vi "MeasurementStatus.vi"(8 "error in (no error)":errorcluster, 10 "Current Measurement Idx":i32, 11 "Measurement Sequence":dbl[](array[numeric])) -> (0 "error out":errorcluster, 2 "Sequence Progress":cluster{i32[], "Y":dbl[]}[](array[cluster]))   [LabVIEW 2014]
panel:
  # "LICENSED MATERIALS – PROPERTY OF IBM\nCopyright IBM Corp. 2016,\nALL RIGHTS RESERVED"
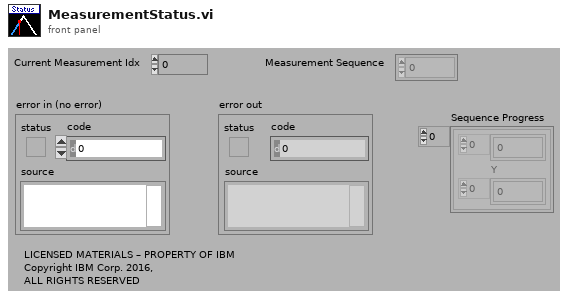
[diagram p1: front panel]
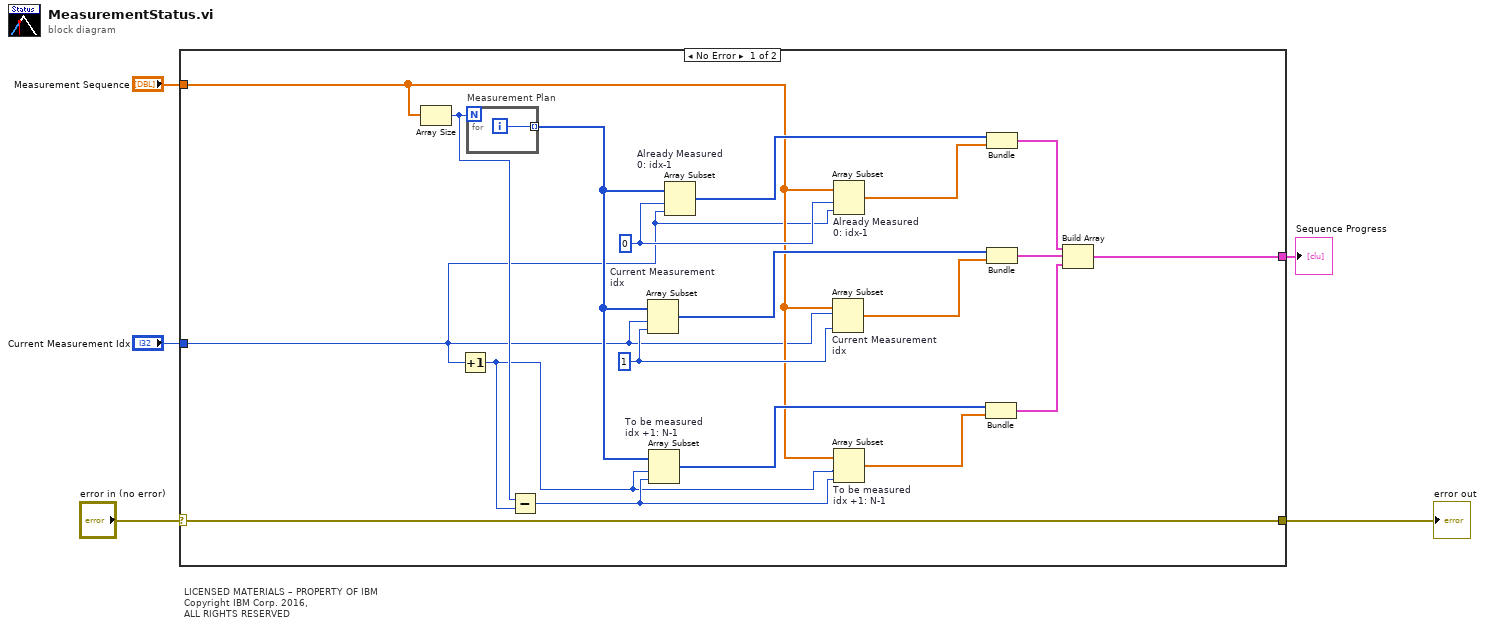
[diagram p0: block diagram]
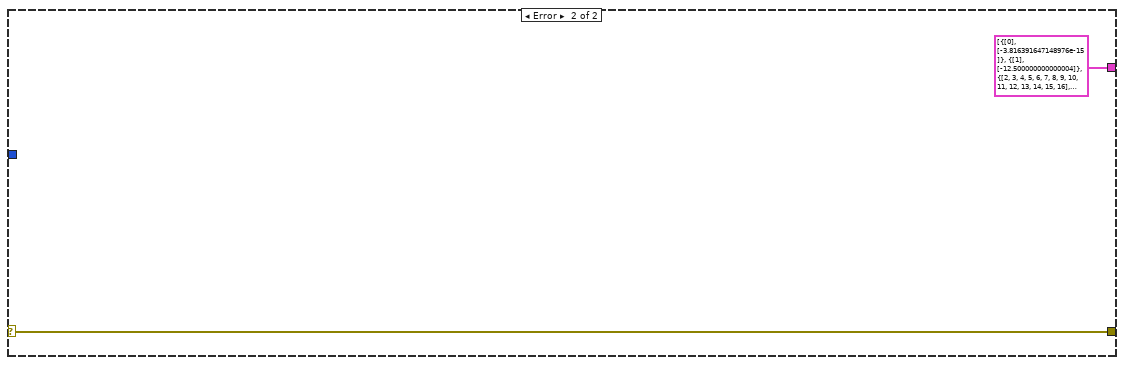
[diagram p2: hidden frame]
diagram:
  # "LICENSED MATERIALS – PROPERTY OF IBM\nCopyright IBM Corp. 2016,\nALL RIGHTS RESERVED"
  n1 = case shown="No Error" "error in (no error)" {
    selector: "error in (no error)" -> [w9 w27]
    tunnel: [w9 w27] -> w4
    tunnel: [w8 cluster{i32[], "Y":dbl[]}[] [{[0], "Y"=[-3.816391647148976e-15]}, {[1], "Y"=[-12.500000000000004]}, {[2, 3, 4, 5, 6, 7, 8, 9, 10, 11, 12, 13, 14, 15, 16], "Y"=[-25.000000000000004, -37.50000000000001, -49.99999999999999, -37.49999999999999, -24.999999999999993, -12.499999999999993, 0.0, 12.5, 25.0, 37.5, 50.0, 37.5, 24.999999999999996, 12.499999999999996, -3.816391647148976e-15]}] ("Sequence Progress 2")] -> w3
    tunnel: "Measurement Sequence" -> [w7 _]
    tunnel: "Current Measurement Idx" -> [w6 _]
    frame No Error {
      w23 = 0 ("index")
      w22 = 1 ("length")
      n2 = Array Size(array=w7) -> (size(s)=w24:i32)
      n3 = Increment(x=w6) -> (x+1=w20:i32)
      n4 = for "Measurement Plan" {
        N: w24 -> [_]
        tunnel: [w25] -> w19 mode=indexing
        i -> [w25]
      }
      n5 = Subtract(x=w24, y=w20) -> (x-y=w21:i32)
      n6 = Array Subset "Current Measurement\nidx"(array=w19, index=w6, length=w22) -> (w16:i32[])
      n7 = Array Subset "To be measured\nidx +1: N-1"(array=w19, index=w20, length=w21) -> (w14:i32[])
      n8 = Array Subset "Already Measured\n0: idx-1"(array=w19, index=w23, length=w6) -> (w18:i32[])
      n9 = Array Subset "Current Measurement\nidx"(array=w7, index=w6, length=w22) -> (w15:dbl[])
      n10 = Array Subset "Already Measured\n0: idx-1"(array=w7, index=w23, length=w6) -> (w17:dbl[])
      n11 = Array Subset "To be measured\nidx +1: N-1"(array=w7, index=w20, length=w21) -> (w13:dbl[])
      n12 = Bundle(w14, w13) -> (w10:cluster{i32[], dbl[]})  [unwired: 1 out]
      n13 = Bundle(w18, w17) -> (w12:cluster{i32[], dbl[]})  [unwired: 1 out]
      n14 = Bundle(w16, w15) -> (w11:cluster{i32[], dbl[]})  [unwired: 1 out]
      n15 = Build Array(w12, w11, w10) -> (w8:cluster{i32[], dbl[]}[])
    }
    frame Error {
    }
  }
  "error out" <- w4
  "Sequence Progress" <- w3
